vi "Write Settings_Ref.vi"(8 "error in":errorcluster, 10 "Settings_Ref":refnum<vi>, 11 "PowerSupply in":refnum<class "PowerSupply.lvclass">) -> (0 "error out":errorcluster, 3 "PowerSupply out":refnum<class "PowerSupply.lvclass">)   [LabVIEW 2019, in "PowerSupply.lvlib" / "PowerSupply.lvclass"]
uses:
  Library/PowerSupply.lvclass
  Custom Controls/Settings.ctl
  Custom Controls/Sense Point.ctl
  Custom Controls/OCP Mode.ctl
  Library/PowerSupply.lvclass/PowerSupply.ctl
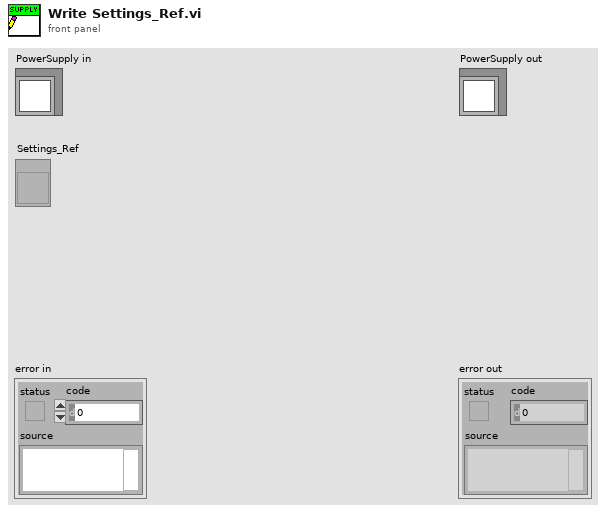
[diagram p1: front panel]
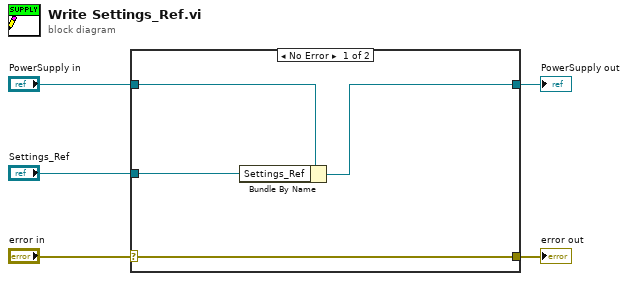
[diagram p0: block diagram]
diagram:
  n1 = case shown="No Error" "error in" {
    selector: "error in" -> [w9 w10]
    tunnel: [w9 w10] -> w4
    tunnel: [w7 w11] -> w2
    tunnel: "PowerSupply in" -> [w8 w11]
    tunnel: "Settings_Ref" -> [w6 _]
    frame No Error {
      n2 = Bundle By Name(cluster=w8, "Settings_Ref"=w6) -> (w7:refnum<class "PowerSupply.lvclass">)
    }
    frame Error {
    }
  }
  "error out" <- w4
  "PowerSupply out" <- w2
